vi "Parse XML String for Multiple Nodes.vi"(10 "XML String":string="<?xml version=\"1.0\" encoding=\"ISO-8859-1\"?>\n<bookstore>\n<book ISBN=\"978-0545128285\">\n  <title lang=\"en\">The Tales of Beedle the Bard</title>\n  <author>J. K. Rowling</author>\n  <year>2008</year>\n  <price>12.99</price>\n</book>\n<book ISBN=\"978-0316160209\">\n  <title lang=\"en\">Eclipse</title>\n  <author>Stephenie Meyer</author>\n  <year>2007</year>\n  <price>19.99</price>\n</book>\n<book ISBN=\"978-0316067928\">\n  <title lang=\"en\">Breaking Dawn</title>\n  <author>Stephenie Meyer</author>\n  <year>2008</year>\n  <price>22.99</price>\n</book>\n<book ISBN=\"978-0316017923\">\n  <title lang=\"en\">Outliers: The Story of Success</title>\n  <author>Malcolm Gladwell</author>\n  <year>2008</year>\n  <price>27.99</price>\n</book>\n<book ISBN=\"978-0596007645\">\n  <title lang=\"en\">XML in a Nutshell</title>\n  <author>Elliotte Rusty Harold</author>\n  <author>W. Scott Means</author>\n  <year>2004</year>\n  <price>39.95</price>\n</book>\n</bookstore>", 11 "XPath Expression":string="/bookstore/book/title") -> (3 "Search Results":string[](array[string]))   [LabVIEW 2015]
doc: "This example demonstrates how to query an XML document by using an XPath expression and returns all the nodes that match the XPath expression."
uses:
  <resource>/objmgr/DOMUserDefRef.rc
  <vilib>/xml/NI_XML.lvlib
  <vilib>/xml/Close Reference(Node).vi
  <vilib>/xml/Load XML String.vi
panel:
  # "Overview: Demonstrates the use of the XML Parser VIs and functions to search an XML string for multiple nodes (tags) that match a given XPath search expression.\nInstructions:\nRun the VI."
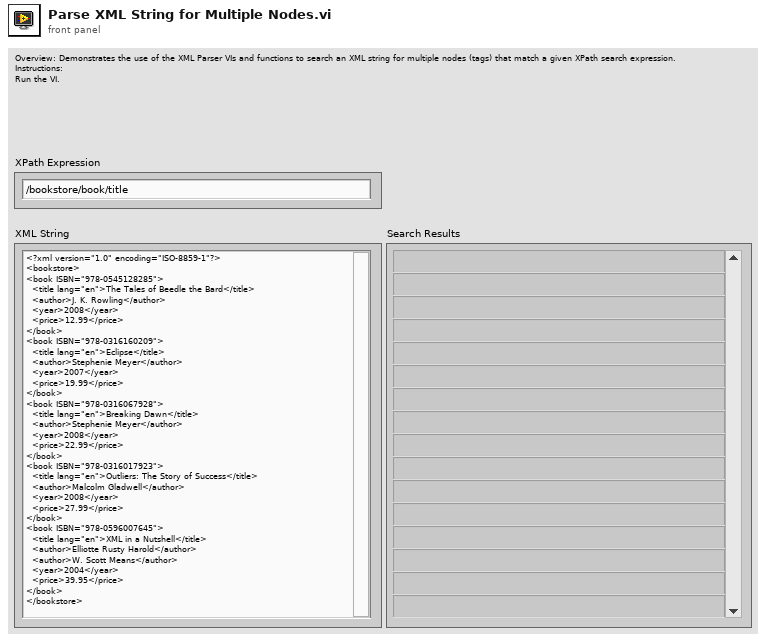
[diagram p1: front panel]
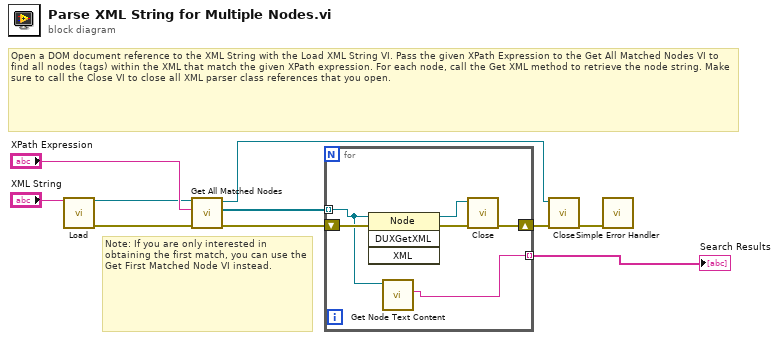
[diagram p0: block diagram]
diagram:
  # "Note: If you are only interested in obtaining the first match, you can use the Get First Matched Node VI instead."
  # "Open a DOM document reference to the XML String with the Load XML String VI. Pass the given XPath Expression to the Get All Matched Nodes VI to find all nodes (tags) within the XML that match the given XPath expression. For each node, call the Get XML method to retrieve the node string. Make sure to call the Close VI to close all XML parser class references that you open."
  n1 = call-poly <vilib>:"Load.vi"("XML string"="XML String") -> ("DOM document out"=w2:refnum<k20>, "error out"=w1:errorcluster)  [unwired: 12 in, 1 out]
  n2 = call <vilib>:"Get All Matched Nodes.vi"("error in (no error)"=w1, "XPath expression"="XPath Expression", "node in"=w2) -> ("error out"=w9:errorcluster, "node result array"=w10:refnum<k20>[], "node out"=w6:refnum<k20>)  [unwired: 6 out]
  n3 = for {
    tunnel: w10 -> [w12] mode=indexing
    shift-right: [w14] -> w7
    shift-left: w9 -> [w13]
    tunnel: [w11] -> w4 mode=indexing
    n4 = invoke on="Invoke Node" class="Node" method="DUXGetXML"(reference=w12, error in=w13) -> (reference out=w15:refnum<k20>, error out=w16:errorcluster)  [unwired: 2 in, 2 out]
    n5 = call <vilib>:"Get Node Text Content.vi"("node in"=w12) -> ("node text"=w11:string)  [unwired: 8 in, 2 out]
    n6 = call-poly <vilib>:"Close.vi"("error in (no error)"=w16, "node"=w15) -> ("error out"=w14:errorcluster)  [unwired: 7 out]
  }
  "Search Results" <- w4
  n7 = call-poly <vilib>:"Close.vi"("error in (no error)"=w7, "node"=w6) -> ("error out"=w5:errorcluster)  [unwired: 7 out]
  n8 = call <vilib>:"Simple Error Handler.vi"("error in (no error)"=w5) -> ()  [unwired: 1 in, 8 out]
